vi "FTW-File-CreateDirectory.vi"(0 "Directory to Create":path, 11 "error in":errorcluster) -> (4 "Created Directory":path, 15 "error out":errorcluster)   [LabVIEW 2015]
panel:
  # "Inputs"
  # "Outputs"
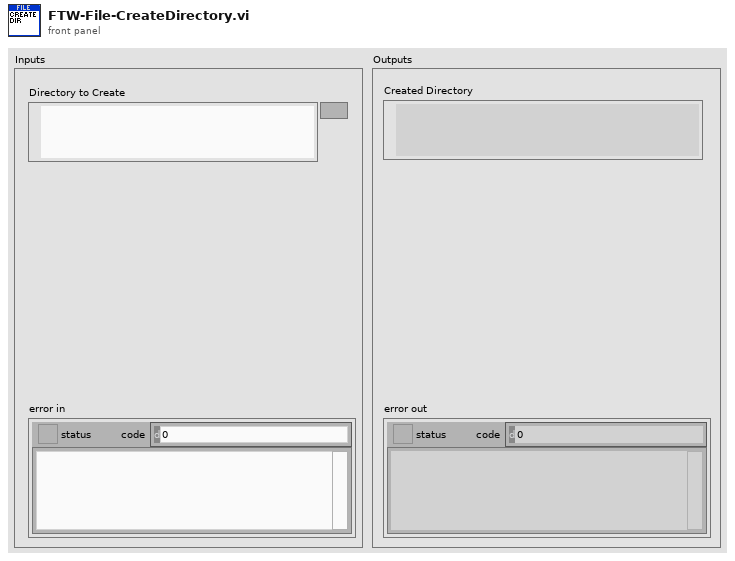
[diagram p1: front panel]
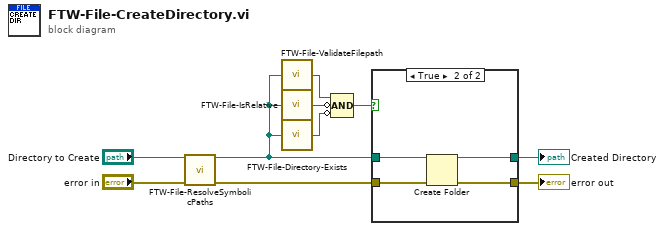
[diagram p0: block diagram]
diagram:
  n1 = call "FTW-File-ResolveSymbolicPaths.vi"("Unresolved Path"="Directory to Create", "error in"="error in") -> ("Resolved Path"=w3:path, "error out"=w1:errorcluster)  [unwired: 12 in]
  n2 = call "FTW-File-ValidateFilepath.vi"("Filepath"=w3) -> ("Valid?"=w8:bool)
  n3 = call "FTW-File-IsRelative.vi"("Filepath"=w3) -> ("Relative?"=w7:bool)
  n4 = call "FTW-File-Directory-Exists.vi"("Directory"=w3) -> ("Exists?"=w6:bool)
  n5 = Compound Arithmetic op=AND(w8, invert w7, invert w6) -> (w5:bool)
  n6 = case shown="True" w5 {
    tunnel: [w12 w16] -> w10
    tunnel: w1 -> [w11 w15]
    tunnel: w3 -> [w12 w14]
    tunnel: [w11 w13] -> w9
    frame False {
    }
    frame True {
      n7 = Create Folder(path (use dialog)=w14, error in=w15) -> (created path=w16:path, error out=w13:errorcluster)  [unwired: 1 in, 1 out]
    }
  }
  "error out" <- w9
  "Created Directory" <- w10
